vi "Read tcp connection.vi"(8 "error in (no error)":errorcluster, 11 "IP Data Unit in":refnum<class "IP Data Unit.lvclass">) -> (0 "error out":errorcluster, 2 "tcp connection":refnum<k5>, 3 "IP Data Unit out":refnum<class "IP Data Unit.lvclass">)   [LabVIEW 2021, in "IP Data Unit.lvclass"]
uses:
  IP Data Unit.lvclass
  IP Data Unit.lvclass/IP Data Unit.ctl
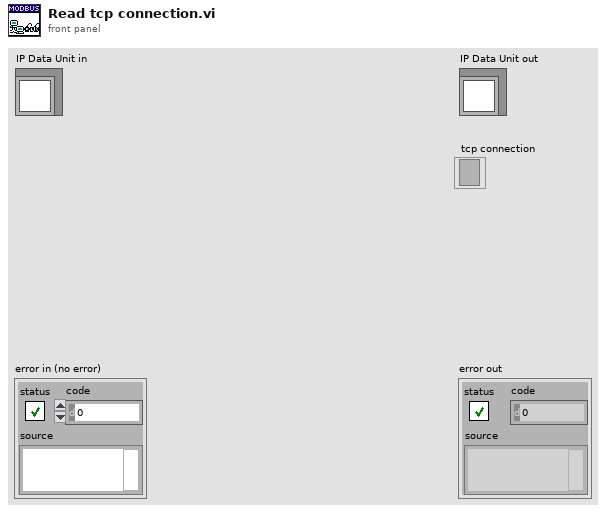
[diagram p1: front panel]
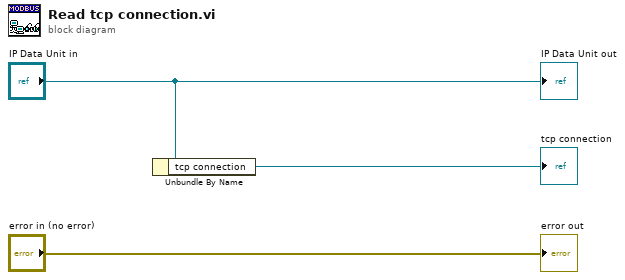
[diagram p0: block diagram]
diagram:
  n1 = Unbundle By Name("IP Data Unit in") -> ("tcp connection"=→"tcp connection":refnum<k5>)
  "error out" <- "error in (no error)"
  "IP Data Unit out" <- "IP Data Unit in"
